vi "Copy Channel.vi"(8 "error in (no error)":errorcluster, 10 "Channel to Receive Copy (1)":dbl=1.0 min=1.0 max=4.0, 11 "VISA resource name":refnum<visa-resource-name>) -> (0 "error out":errorcluster, 3 "VISA resource name out":refnum<visa-resource-name>)   [LabVIEW 2015, in "Fluke 28x Series.lvlib"]
doc: "Copies the current channel's details over into the channel specified by <b>Channel to Receive Copy</b>.\n\n<b>Note</b>: This VI applies only to multichannel instruments, i.e. Fluke 282 and Fluke 284."
uses:
  <instrlib>/Fluke 28x Series/Fluke 28x Series.lvlib
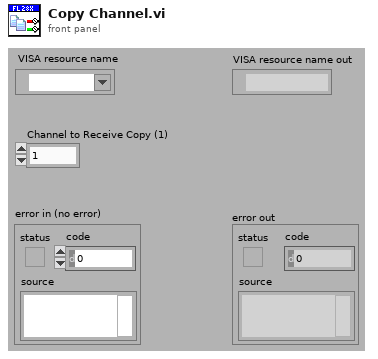
[diagram p1: front panel]
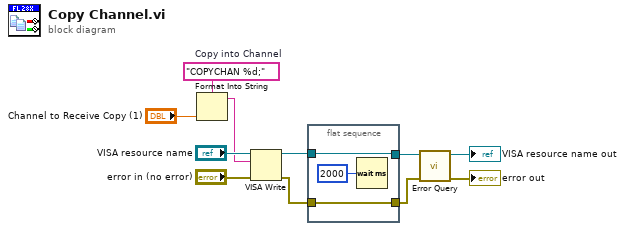
[diagram p0: block diagram]
diagram:
  w10 = "COPYCHAN %d;"  # Copy into Channel
  n1 = Format Into String(format string=w10, "Channel to Receive Copy (1)") -> (resulting string=w7:string)  [unwired: 2 in, 1 out]
  n2 = VISA Write(VISA resource name="VISA resource name", write buffer=w7, error in (no error)="error in (no error)") -> (VISA resource name out=w4:refnum<visa-resource-name>, error out=w2:errorcluster)  [unwired: 1 out]
  n3 = flat-sequence {
    tunnel: [w13] -> w3
    tunnel: w4 -> [w13]
    tunnel: w2 -> [w12]
    tunnel: [w12] -> w1
    frame #0 {
      n4 = Wait (ms)(milliseconds to wait=u32 2000) -> ()  [unwired: 1 out]
    }
  }
  n5 = call <instrlib>:"Error Query.vi"("error in (no error)"=w1, "VISA resource name"=w3) -> ("error out"=→"error out":errorcluster, "VISA resource name out"=→"VISA resource name out":refnum<visa-resource-name>)  [unwired: 6 in, 2 out]
